vi "uTTA_Memory_Writetest.vi"(4 "error in":errorcluster, 7 "VISA Refnum in":refnum<visa-resource-name>) -> (0 "error out":errorcluster, 2 "Received":string, 3 "VISA Refnum out":refnum<visa-resource-name>)   [LabVIEW 2021]
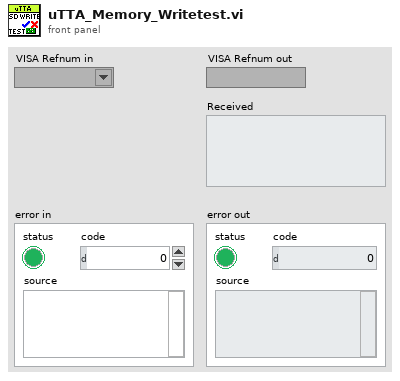
[diagram p1: front panel]
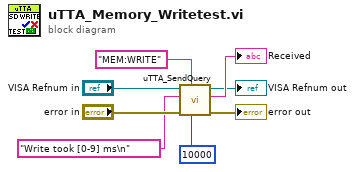
[diagram p0: block diagram]
diagram:
  n1 = call "uTTA_SendQuery.vi"("Timeout(ms)"=10000, "Send String"="MEM:WRITE" ("format string"), "error in (no error)"="error in", "TX Termination(\\n)"="Write took [0-9] ms\n" ("RX Termination(\\n)"), "VISA Refnum in"="VISA Refnum in") -> ("error out"=→"error out":errorcluster, "Received"=→"Received":string, "VISA Refnum out"=→"VISA Refnum out":refnum<visa-resource-name>)  [unwired: 4 in]
